vi "publishEvent.vi"() -> ()   [LabVIEW 2016]
uses:
  ts_sallv_exa/DataTypes/SummaryState.ctl
  ts_sallv_exa/DataTypes/logevent_summaryState.ctl
  SystemSettings/SystemSettings.lvclass
  ts_sallv_exa/SALLV_EXA.lvlib
panel:
  in  "error in (no error)":errorcluster
  out "error out":errorcluster
  in  "SummaryState":T1=enum."DisabledState"
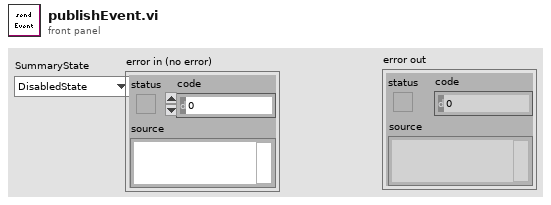
[diagram p1: front panel]
types:
  T1 = typedef "SALLV_EXA.lvlib/SummaryState.ctl" = enum32{"", "DisabledState", "EnabledState", "FaultState", "OfflineState", "StandbyState"}
  T2 = typedef "SALLV_EXA.lvlib/logevent_summaryState.ctl" = cluster{"summaryState":i32, "priority":i32}
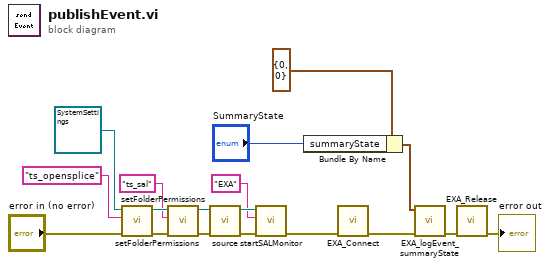
[diagram p0: block diagram]
diagram:
  n1 = call "setFolderPermissions.vi"("error in (no error)"="error in (no error)", "Folder"="ts_opensplice" ("command line"), "SystemSettings in"=refnum<class "SystemSettings.lvclass"> refnum) -> ("error out"=w9:errorcluster, "SystemSettings out"=w8:refnum<class "SystemSettings.lvclass">)  [unwired: 7 in]
  n2 = call "setFolderPermissions.vi"("error in (no error)"=w9, "Folder"="ts_sal" ("command line"), "SystemSettings in"=w8) -> ("error out"=w6:errorcluster, "SystemSettings out"=w5:refnum<class "SystemSettings.lvclass">)  [unwired: 7 in]
  n3 = call "source.vi"("error in (no error)"=w6, "SystemSettings in"=w5) -> ("error out"=w2:errorcluster, "SystemSettings out"=w4:refnum<class "SystemSettings.lvclass">)  [unwired: 8 in]
  n4 = call "startSALMonitor.vi"("error in (no error)"=w2, "Component"="EXA", "SystemSettings in"=w4) -> ("error out"=w1:errorcluster)  [unwired: 7 in, 1 out]
  n5 = Bundle By Name(cluster=T2 {"summaryState"=0, "priority"=0} ("logevent_summaryState_Ctl"), "summaryState"="SummaryState") -> (w16:T2)
  n6 = call "EXA_Connect.vi"("error in (no error)"=w1) -> ("error out"=w14:errorcluster)  [unwired: 9 in, 1 out]
  n7 = call "EXA_logEvent_summaryState.vi"("error in (no error)"=w14, "logevent_summaryState_Ctl"=w16) -> ("error out"=w15:errorcluster)  [unwired: 7 in, 2 out]
  n8 = call "EXA_Release.vi"("error in (no error)"=w15) -> ("error out"=→"error out":errorcluster)  [unwired: 9 in, 1 out]
